vi "Add Resource (File).vi"(8 "error in (no error)":errorcluster, 9 "description":string, 10 "file path":path, 11 "server id":i32) -> (0 "error out":errorcluster, 3 "server id out":i32)   [LabVIEW 2020, in "MCP Server.lvlib"]
doc: "Adds a resource to a MCP server. Resources are files or information (text) that can be added to a prompt by a user in the client similar to a prompt. A Resource does not have parameters and usually returns a file (txt, md, pdf, png).\n\nThis adds a file that will be fully retrieved. Make sure not so exceed several MB of file size.\nSupported file types: text files, pdf, png"
uses:
  MCP Server.lvlib
  resource data.ctl
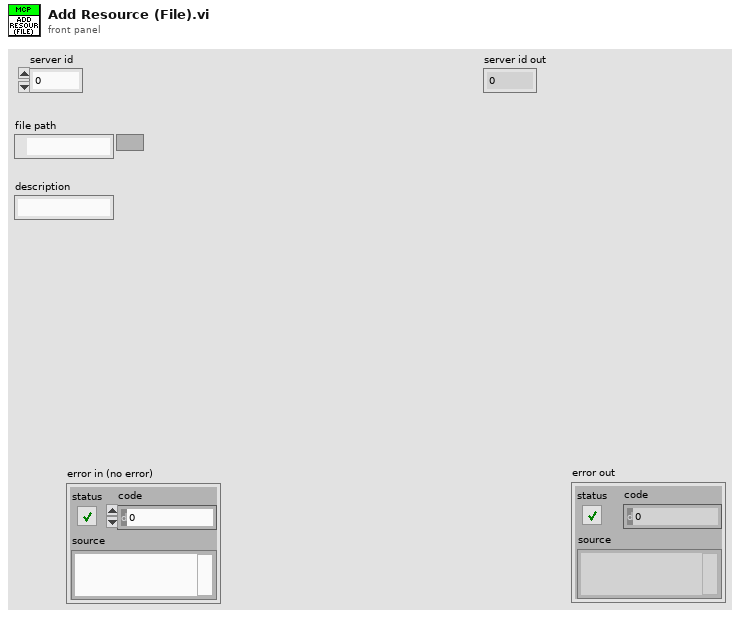
[diagram p1: front panel]
types:
  T1 = typedef "MCP Server.lvlib/resource data.ctl" = cluster{"uri":string, "name":string, "description":string, "mimeType":string, "file path":path}
  T2 = typedef "MCP Server.lvlib/Server Data.ctl" = cluster{"Name":string, "Description":string, "Tools":T3[], "Parameters":string[][], "Logging Info":T6, "User Events":T7, "Prompts":T8[], "resources":T1[], "HTTP Server":refnum<class "Server.lvclass">}
  T3 = typedef "MCP Server.lvlib/Tool Data.ctl" = cluster{"Name":string, "Description":string, "Ignored":string[], "inputs":T4[], "outputs":T5[], "VI Refnum":refnum<vi>}
  T4 = typedef "MCP Server.lvlib/Input Parameter.ctl" = cluster{"name":string, "type":string, "description":string, "required":bool, "raw name":string}
  T5 = typedef "MCP Server.lvlib/Output Parameter.ctl" = cluster{"name":string, "description":string, "type":string, "raw name":string}
  T6 = typedef "MCP Server.lvlib/Logging.ctl" = cluster{"Log":string[], "Max Length":i32}
  T7 = typedef "MCP Server.lvlib/User Events.ctl" = cluster{"onError":refnum<user-event>, "onRpc":refnum<user-event>}
  T8 = typedef "MCP Server.lvlib/Prompt Data.ctl" = cluster{"name":string, "description":string, "arguments":T9[], "return terminal name":string, "results description":string, "VI Refnum":refnum<vi>}
  T9 = typedef "MCP Server.lvlib/Prompt Argument.ctl" = cluster{"name":string, "description":string, "required":bool, "raw_name":string}
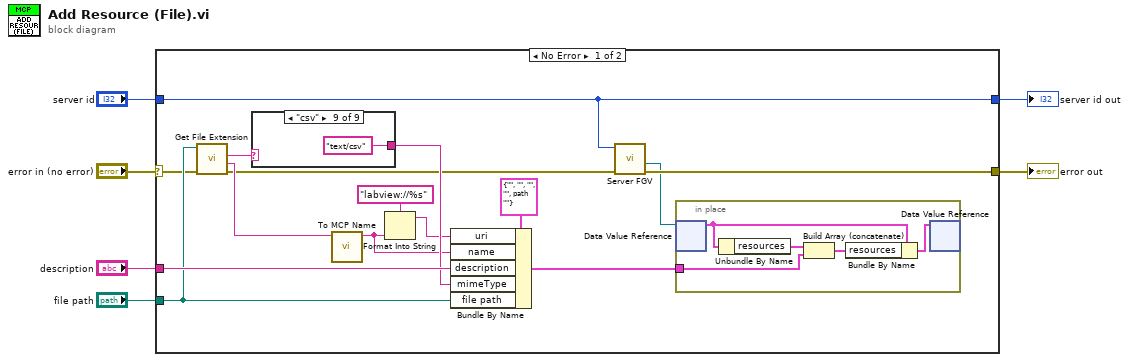
[diagram p0: block diagram]
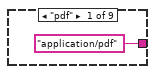
[diagram p2: hidden frame]
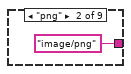
[diagram p3: hidden frame]
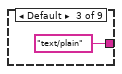
[diagram p4: hidden frame]
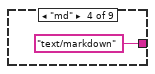
[diagram p5: hidden frame]
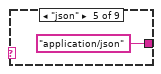
[diagram p6: hidden frame]
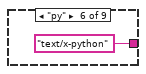
[diagram p7: hidden frame]
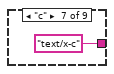
[diagram p8: hidden frame]
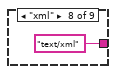
[diagram p9: hidden frame]
diagram:
  n1 = case shown="No Error" "error in (no error)" {
    selector: "error in (no error)" -> [w8 w37]
    tunnel: [w21 w37] -> w6
    tunnel: "server id" -> [w7 w36]
    tunnel: "description" -> [w16 _]
    tunnel: "file path" -> [w12 _]
    tunnel: [w7 w36] -> w1
    frame No Error {
      n2 = call <vilib>:"Get File Extension.vi"("error in (no error)"=w8, "file"=w12) -> ("error out"=w13:errorcluster, "filename without extension"=w19:string, "lowercase file extension"=w15:string)  [unwired: 5 in, 2 out]
      n3 = case shown="\"csv\"" w15 {
        tunnel: ["application/pdf" ("mimeType") "image/png" ("mimeType") "text/plain" ("mimeType") "text/markdown" ("mimeType") "application/json" ("mimeType") "text/x-python" ("mimeType") "text/x-c" ("mimeType") "text/xml" ("mimeType") "text/csv" ("mimeType")] -> w14
        frame "pdf" {
        }
        frame "png" {
        }
        frame Default {
        }
        frame "md" {
        }
        frame "json" {
        }
        frame "py" {
        }
        frame "c" {
        }
        frame "xml" {
        }
        frame "csv" {
        }
      }
      n4 = call "To MCP Name.vi"("unformatted name"=w19) -> ("MCP name"=w9:string)  [unwired: 10 in]
      n5 = Format Into String(format string="labview://%s", w9) -> (resulting string=w11:string)  [unwired: 2 in, 1 out]
      n6 = Bundle By Name(cluster=T1 {"uri"="", "name"="", "description"="", "mimeType"="", "file path"=path ""}, "uri"=w11, "name"=w9, "description"=w16, "mimeType"=w14, "file path"=w12) -> (w17:T1)
      n7 = call "Server FGV.vi"("error in"=w13, "id"=w7) -> ("error out"=w21:errorcluster, "server reference"=w20:refnum<data-value>)  [unwired: 5 in, 3 out]
      n8 = in-place {
        in-place-border: w17 -> [w31]
        n9 = in-place-dvr #1(w20) -> (w34:T2)  [unwired: 1 out]
        n10 = Unbundle By Name(w34) -> ("resources"=w33:T1[])
        n11 = Build Array (concatenate)(w33, w31) -> (w32:T1[])
        n12 = Bundle By Name(cluster=w34, "resources"=w32) -> (w35:T2)
        n13 = in-place-dvr #1(w35) -> ()  [unwired: 2 out]
      }
    }
    frame Error {
    }
  }
  "error out" <- w6
  "server id out" <- w1
